vi "test.vi"() -> ()   [LabVIEW 2016]
panel:
  out "Waveform Chart":dbl(graph)
  out "AI2":dbl
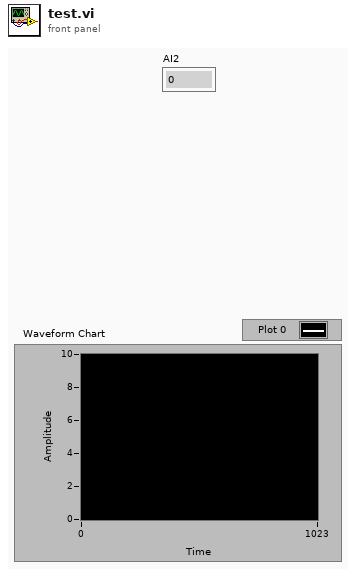
[diagram p1: front panel]
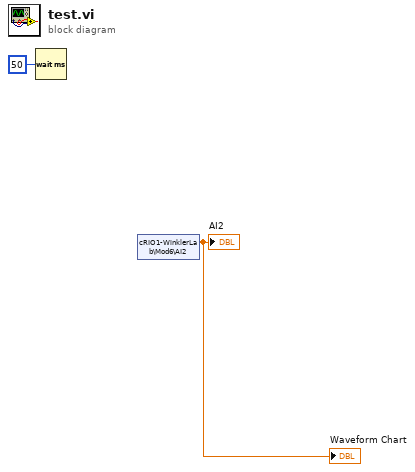
[diagram p0: block diagram]
diagram:
  n1 = Wait (ms)(milliseconds to wait=u32 50) -> ()  [unwired: 1 out]
  n2 = shared-variable "cRIO1-WinklerLab\\Mod6\\AI2"() -> (→"AI2" →"Waveform Chart":dbl)  [unwired: 1 in, 1 out]
